vi "GetFreeFields.vi"(8 "error in (no error)":errorcluster, 11 "SnakeGame in":refnum<class "SnakeGame.lvclass">) -> (0 "error out":errorcluster, 2 "FreeFields":cluster{i16, i16}[](array[cluster]), 3 "SnakeGame out":refnum<class "SnakeGame.lvclass">)   [LabVIEW 2019, in "RT_Game.lvlib" / "SnakeGame.lvclass"]
uses:
  SnakeGame.lvclass
  SnakeGame.lvclass/SnakeGame.ctl
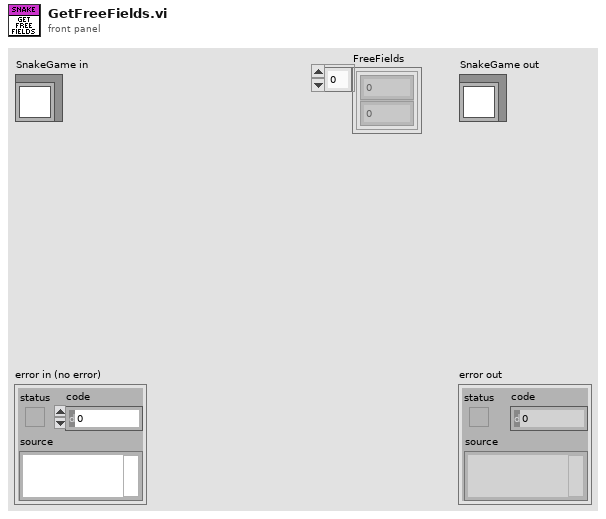
[diagram p1: front panel]
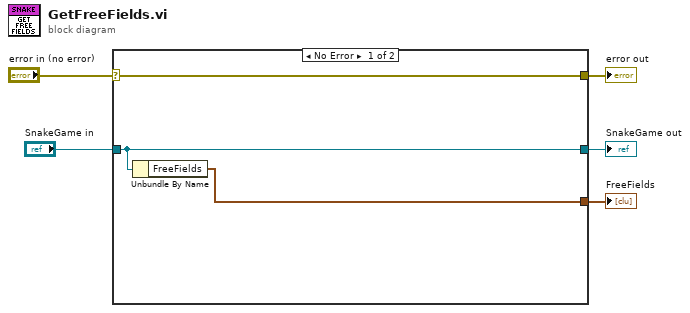
[diagram p0: block diagram]
diagram:
  n1 = case shown="No Error" "error in (no error)" {
    selector: "error in (no error)" -> [w8 w10]
    tunnel: [w8 w10] -> w4
    tunnel: [w7 w9] -> w2
    tunnel: "SnakeGame in" -> [w7 w9]
    tunnel: [w6 _] -> w1
    frame No Error {
      n2 = Unbundle By Name(w7) -> ("FreeFields"=w6:cluster{"x":i16, "y":i16}[])
    }
    frame Error {
    }
  }
  "error out" <- w4
  "SnakeGame out" <- w2
  "FreeFields" <- w1
